vi "sv_Set Next Circular Buffer Index.vi"(8 "read/write indices":T1(array[cluster]), 10 "current index":i32) -> (2 "new index":i32)   [LabVIEW 2017, in "SoundVib_SweptSine.lvlib"]
uses:
  <vilib>/addons/Sound and Vibration/svt_Swept Sine/SoundVib_SweptSine.lvlib
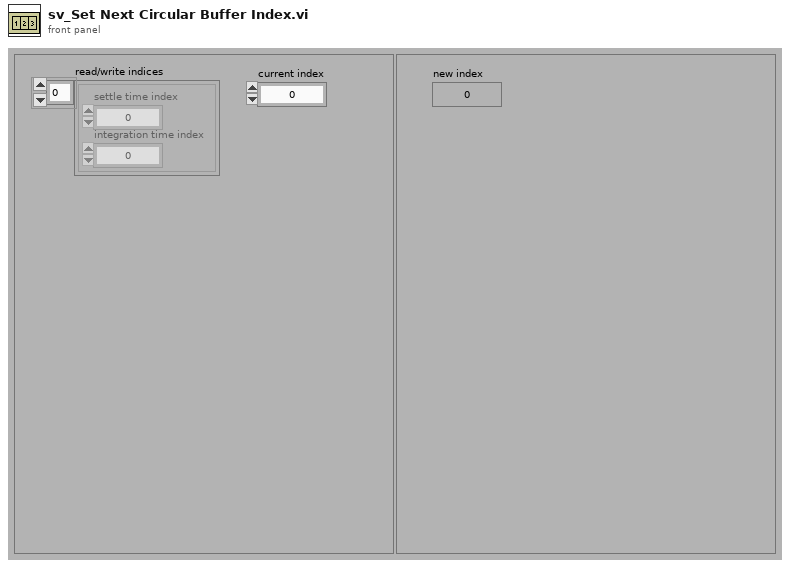
[diagram p1: front panel]
types:
  T1 = cluster{"settle time index":u32, "integration time index":u32}[]
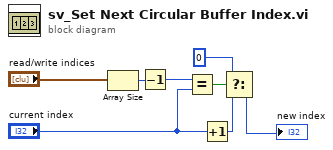
[diagram p0: block diagram]
diagram:
  n1 = Array Size(array="read/write indices") -> (size(s)=w3:i32)
  n2 = Decrement(x=w3) -> (x-1=w8:i32)
  n3 = Equal?(x=w8, y="current index") -> (x = y?=w4:bool)
  n4 = Increment(x="current index") -> (x+1=w5:i32)
  n5 = Select(t=0, s=w4, f=w5) -> (s? t:f=→"new index":i32)
